vi "Borders and Shading Constant Shell.vi"   [LabVIEW 2020]
doc: "Defines the borders and shading attributes of a document."
uses:
  <vilib>/addons/_office/NI_ReportGenerationToolkit.lvlib
types:
  T1 = cluster{"OutsideLineStyle":i32, "OutsideColorIndex":u32, "OutsideLineWidth":i32, "BackgroundPatternColor":u32}
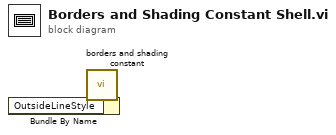
[diagram p0: block diagram]
diagram:
  n1 = call <vilib>:"borders and shading constant.vi"() -> ("borders and shading"=w1:T1)
  n2 = Bundle By Name(cluster=w1) -> ()  [unwired: 1 in, 1 out]
